vi "Create Simulated Detector.vi"(8 "error in (no error)":errorcluster, 9 "Event Threshold (0-1)":dbl, 10 "Master":bool, 11 "Name":string) -> (0 "error out":errorcluster, 3 "Simulated Detector out":refnum<class "Simulated Detector.lvclass">)   [LabVIEW 2019, in "Simulated Detector.lvclass"]
uses:
  Simulated Detector.lvclass
  Simulated Detector.lvclass/Simulated Detector.ctl
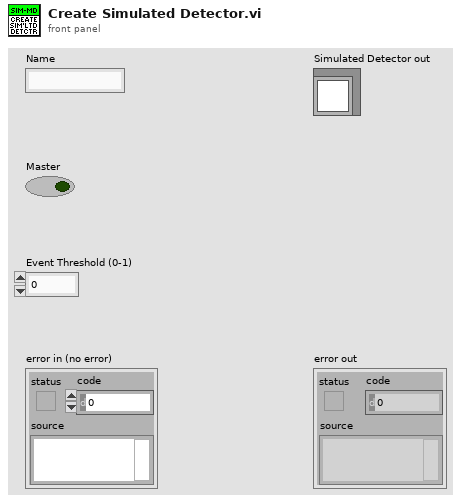
[diagram p1: front panel]
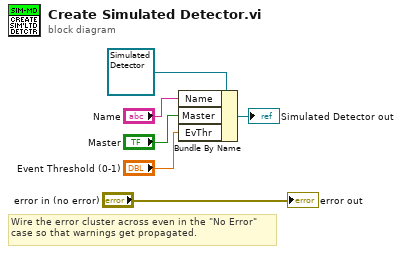
[diagram p0: block diagram]
diagram:
  # "Wire the error cluster across even in the \"No Error\"\ncase so that warnings get propagated."
  n1 = Bundle By Name(cluster=refnum<class "Simulated Detector.lvclass"> refnum ("Simulated Detector in"), "Name"="Name", "Master"="Master", "EvThr"="Event Threshold (0-1)") -> (→"Simulated Detector out":refnum<class "Simulated Detector.lvclass">)
  "error out" <- "error in (no error)"
